vi "check-tool-done.vi"(11 "Subsystem in":string) -> ()   [LabVIEW 2017]
uses:
  automode-scripting.lvlib
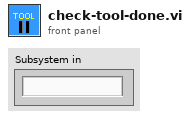
[diagram p1: front panel]
types:
  T1 = enum16{"Add to sent", "Add to complete", "Get arrays"}
  T2 = typedef "labview-standard-library.lvlib/automode-scripting.lvlib/subsystems.ctl" = string
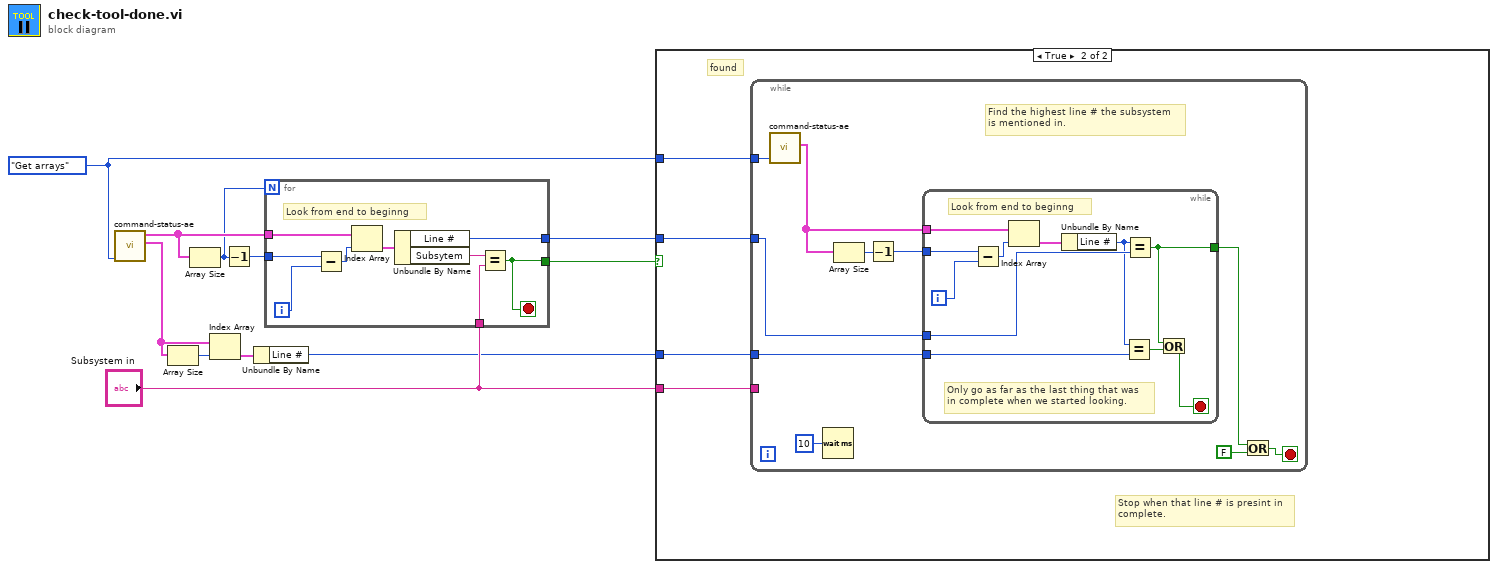
[diagram p0: block diagram]
diagram:
  w11 = T1."Get arrays" ("Engine state")
  n1 = call "command-status-ae.vi"("Engine state"=w11) -> ("Complete"=w2:cluster{"Subsytem":T2, "Line #":i32}[], "Sent"=w9:cluster{"Subsytem":T2, "Line #":i32}[])  [unwired: 9 in]
  n2 = Array Size(array=w2) -> (size(s)=w3:i32)
  n3 = Array Size(array=w9) -> (size(s)=w7:i32)
  n4 = Index Array(array=w2, index=w3) -> (element=w4:cluster{"Subsytem":T2, "Line #":i32})
  n5 = Decrement(x=w7) -> (x-1=w8:i32)
  n6 = Unbundle By Name(w4) -> ("Line #"=w1:i32)
  n7 = for {
    N: w7 -> [_]
    tunnel: w9 -> [w20]
    tunnel: [w18] -> w10
    tunnel: w8 -> [w17]
    tunnel: [w15] -> w6
    tunnel: "Subsystem in" -> [w13]
    i -> [w16]
    stop <- w15 stop-if-true
    # "Look from end to beginng"
    n8 = Subtract(x=w17, y=w16) -> (x-y=w12:i32)
    n9 = Index Array(array=w20, index=w12) -> (element=w19:cluster{"Subsytem":T2, "Line #":i32})
    n10 = Unbundle By Name(w19) -> ("Line #"=w18:i32, "Subsytem"=w14:T2)
    n11 = Equal?(x=w14, y=w13) -> (x = y?=w15:bool)
  }
  n12 = case shown="True" w6 {
    tunnel: w11 -> [_ w24]
    tunnel: "Subsystem in" -> [_ w23]
    tunnel: w10 -> [_ w22]
    tunnel: w1 -> [_ w21]
    frame False {
      # "Queue to invalid"
      # "Not fount"
    }
    frame True {
      # "Stop when that line # is presint in\ncomplete."
      # "found"
      n13 = while {
        tunnel: w24 -> [w34]
        tunnel: w23 -> [_]
        tunnel: w22 -> [w29]
        tunnel: w21 -> [w30]
        stop <- w28 stop-if-true
        # "Find the highest line # the subsystem\nis mentioned in."
        n14 = call "command-status-ae.vi"("Engine state"=w34) -> ("Complete"=w31:cluster{"Subsytem":T2, "Line #":i32}[])  [unwired: 9 in, 1 out]
        n15 = Wait (ms)(milliseconds to wait=u32 10) -> ()  [unwired: 1 out]
        n16 = Array Size(array=w31) -> (size(s)=w25:i32)
        n17 = Decrement(x=w25) -> (x-1=w32:i32)
        n18 = while {
          tunnel: w31 -> [w45]
          tunnel: w32 -> [w43]
          tunnel: [w41] -> w27
          tunnel: w30 -> [w36]
          tunnel: w29 -> [w39]
          i -> [w42]
          stop <- w35 stop-if-true
          # "Only go as far as the last thing that was\nin complete when we started looking."
          # "Look from end to beginng"
          n19 = Subtract(x=w43, y=w42) -> (x-y=w40:i32)
          n20 = Index Array(array=w45, index=w40) -> (element=w44:cluster{"Subsytem":T2, "Line #":i32})
          n21 = Unbundle By Name(w44) -> ("Line #"=w37:i32)
          n22 = Equal?(x=w37, y=w36) -> (x = y?=w38:bool)
          n23 = Equal?(x=w37, y=w39) -> (x = y?=w41:bool)
          n24 = Or(x=w41, y=w38) -> (x .or. y?=w35:bool)
        }
        n25 = Or(x=w27, y=FALSE) -> (x .or. y?=w28:bool)
      }
    }
  }
